vi "ParamsComposto - Copy.vi"(2 "paramsIn":variant) -> (16 "paramsOut":variant)   [LabVIEW 2017]
uses:
  Typedefs/Tipo_ComponenteSinalComposto.ctl
  Typedefs/Tipo_ParamsComposto.ctl
  Typedefs/Tipo_ComponenteSinalRuidoComposto.ctl
panel:
  in  "Componentes":T1[](array[typedef])=[{"Amplit.: "=0.0, "Freq. (Hz): "=0.0, "Fase (º):"=0.0, "Ruido:"=0.0}, {"Amplit.: "=0.0, "Freq. (Hz): "=0.0, "Fase (º):"=0.0, "Ruido:"=0.0}, {"Amplit.: "=0.0, "Freq. (Hz): "=0.0, "Fase (º):"=0.0, "Ruido:"=0.0}, {"Amplit.: "=0.0, "Freq. (Hz): "=0.0, "Fase (º):"=0.0, "Ruido:"=0.0}]
  in  "Modulation":dbl
  in  "Carrier Frequency":dbl
  in  "Ruído Total":dbl
  in  "Init":bool
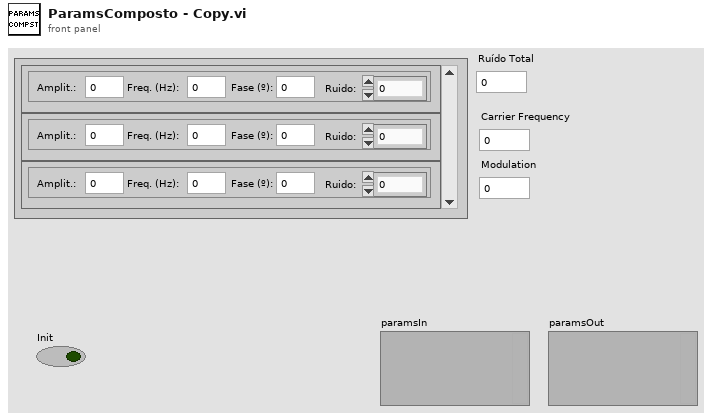
[diagram p1: front panel]
types:
  T1 = typedef "Tipo_ComponenteSinalRuidoComposto.ctl" = cluster{"Amplit.: ":dbl, "Freq. (Hz): ":dbl, "Fase (º):":dbl, "Ruido:":dbl}
  T2 = typedef "Tipo_ParamsComposto.ctl" = cluster{"Componentes":T3[], "Ruído":dbl}
  T3 = typedef "Tipo_ComponenteSinalComposto.ctl" = cluster{"Amplit.: ":dbl, "Freq. (Hz): ":dbl, "Fase (º):":dbl}
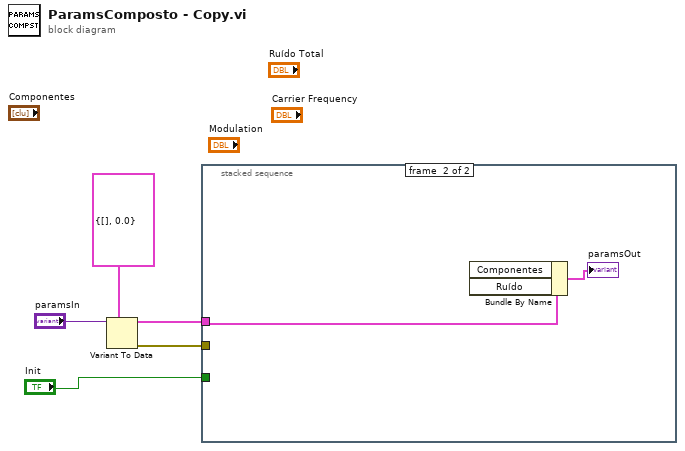
[diagram p0: block diagram]
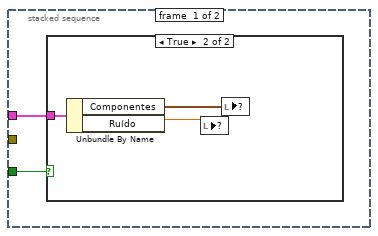
[diagram p2: hidden frame]
diagram:
  n1 = Variant To Data(type=T2 {"Componentes"=[], "Ruído"=0.0}, Variant="paramsIn") -> (data=w4:T2, error out=w2:errorcluster)  [unwired: 1 in]
  n2 = stacked-sequence {
    tunnel: w4 -> [w7 w14]
    tunnel: "Init" -> [w6 _]
    tunnel: w2 -> [_ _]
    frame #0 {
      n3 = case shown="True" w6 {
        tunnel: w7 -> [_ w10]
        frame False {
        }
        frame True {
          n4 = Unbundle By Name(w10) -> ("Componentes"=w9:T3[], "Ruído"=w8:dbl)
          n5 = local write item#-1(w8) -> ()
          n6 = local write item#-1(w9) -> ()
        }
      }
    }
    frame #1 {
      n7 = Bundle By Name(cluster=w14) -> (→"paramsOut":T2, "Componentes"=w11:T3[], "Ruído"=w12:dbl)
    }
  }
